vi "Field_Dist_Pixel_Const.vi"() -> (1 "Y Conv":dbl, 3 "X Conv":dbl)   [LabVIEW 2019]
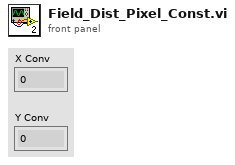
[diagram p1: front panel]
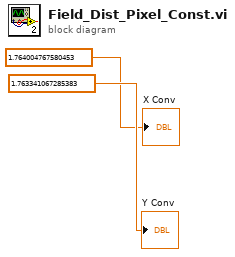
[diagram p0: block diagram]
diagram:
  "Y Conv" <- 1.763341067285383
  "X Conv" <- 1.764004767580453
